vi "loadSettingsFile.vi"(8 "error in (no error)":errorcluster, 10 "Path":path, 11 "CameraManager in":refnum<class "CameraManager.lvclass">) -> (0 "error out":errorcluster, 3 "CameraManager out":refnum<class "CameraManager.lvclass">)   [LabVIEW 2009, in "iManagement.lvlib" / "CameraManager.lvclass"]
doc: "Load the camera settings from the camera settings file xml."
uses:
  CameraManager.lvclass
  CameraManager.lvclass/CameraManager.ctl
  Hal/Channels/Camera/CameraController.lvclass
  Hal/Channels/Camera/CameraEventsManager/CameraEventsManger.lvclass
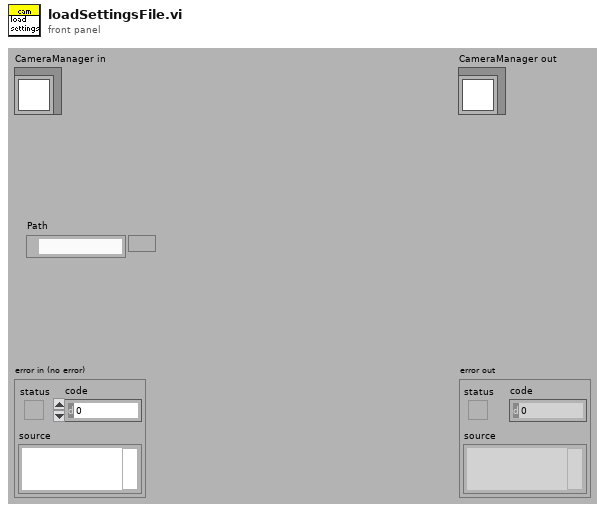
[diagram p1: front panel]
types:
  T1 = cluster{"settingsFrontEndEvents":cluster{"loadSettingsFromPath":refnum<user-event>, "lookUpElementEvent":refnum<user-event>, "saveSettings":refnum<user-event>, "loadSettings":refnum<user-event>, "close":refnum<user-event>, "replaceElement":refnum<user-event>, "findParentNodes":refnum<user-event>, "createNode":refnum<user-event>}, "settingBackEndEvents":cluster{"defaultSettingsPathRequest":refnum<user-event>, "searchResultEvent":refnum<user-event>, "settingsSaved":refnum<user-event>, "settingsLoaded":refnum<user-event>, "foundParentNode":refnum<user-event>}}
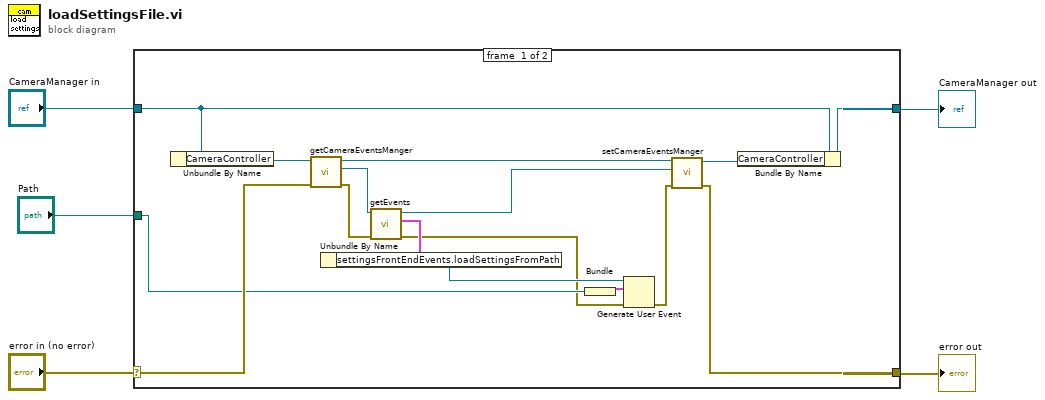
[diagram p0: block diagram]
diagram:
  n1 = case shown="No Error" "error in (no error)" {
    selector: "error in (no error)" -> [w14 w23]
    tunnel: [w6 w23] -> w4
    tunnel: [w15 w22] -> w2
    tunnel: "CameraManager in" -> [w18 w22]
    tunnel: "Path" -> [w10 _]
    frame #0 {
      n2 = Unbundle By Name(w18) -> ("CameraController"=w19:refnum<class "CameraController.lvclass">)
      n3 = call-dynamic "getCameraEventsManger.vi"("error in (no error)"=w14, "CameraController.lvclass in"=w19) -> ("error out"=w20:errorcluster, "Hardware:Channels.lvlib:CameraEventsManger.lvclass"=w21:refnum<class "CameraEventsManger.lvclass">, "CameraController.lvclass out"=w17:refnum<class "CameraController.lvclass">)  [unwired: 7 in]
      n4 = call-dynamic "getEvents.vi"("error in (no error)"=w20, "CameraEventsManger in"=w21) -> ("error out"=w8:errorcluster, "settingsEvents"=w12:T1, "CameraEventsManger out"=w13:refnum<class "CameraEventsManger.lvclass">)  [unwired: 5 in, 2 out]
      n5 = Unbundle By Name(w12) -> ("settingsFrontEndEvents.loadSettingsFromPath"=w11:refnum<user-event>)
      n6 = Bundle("Path"=w10) -> (w9:cluster{"Path":path})  [unwired: 1 in]
      n7 = Generate User Event(user event=w11, event data cluster=w9, error in=w8) -> (error out=w7:errorcluster)  [unwired: 1 out]
      n8 = call-dynamic "setCameraEventsManger.vi"("error in (no error)"=w7, "Hardware:Channels.lvlib:CameraEventsManger.lvclass"=w13, "CameraController.lvclass in"=w17) -> ("error out"=w6:errorcluster, "CameraController.lvclass out"=w16:refnum<class "CameraController.lvclass">)  [unwired: 7 in]
      n9 = Bundle By Name(cluster=w18, "CameraController"=w16) -> (w15:refnum<class "CameraManager.lvclass">)
    }
    frame #1 {
    }
  }
  "error out" <- w4
  "CameraManager out" <- w2
